vi "Chuck Has Pottable Modules.vi"(8 "error in":errorcluster, 10 "Chuck":i32, 11 "WorkTable in":refnum<class "WorkTable Class.lvclass">=refnum) -> (0 "error out":errorcluster, 2 "Has Pottable Modules":bool, 3 "WorkTable out":refnum<class "WorkTable Class.lvclass">)   [LabVIEW 2017]
uses:
  Shared Components/WorkTable Class/WorkTable Class.lvclass
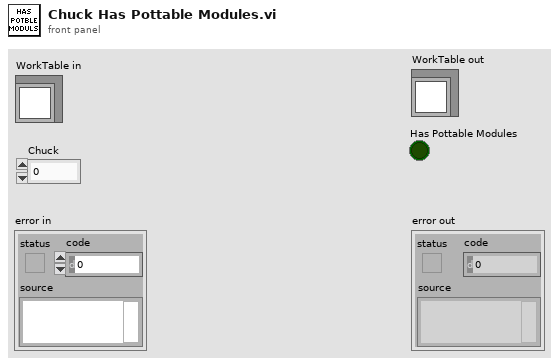
[diagram p1: front panel]
types:
  T1 = typedef "Worktable_Module Slot.ctl" = cluster{"Slot State":enum16{"Empty", "Bare HDI", "Unglued", "Stamped", "PartOnTop", "Weighted", "Unpotted", "Potted"}, "BBM Type":enum16{"None", "BBM", "GlassSlide"}, "HDI Type":enum16{"None", "HDI", "Polyimide"}, "Vacuum Channel":u8, "Location/Orientation BBM":T2, "Location/Orientation HDI":T2, "S/N":string}
  T2 = typedef "Position_Orientation.ctl" = cluster{"Center":refnum<class "Vec3d Class.lvclass">, "Orientation":refnum<class "Orient3d Class.lvclass">}
  T3 = enum16{"Empty", "Unglued", "Stamped", "PartOnTop", "Weighted", "Unpotted", "Potted"}
  T4 = enum16{"Empty", "Bare HDI", "Unglued", "Stamped", "PartOnTop", "Weighted", "Unpotted", "Potted"}
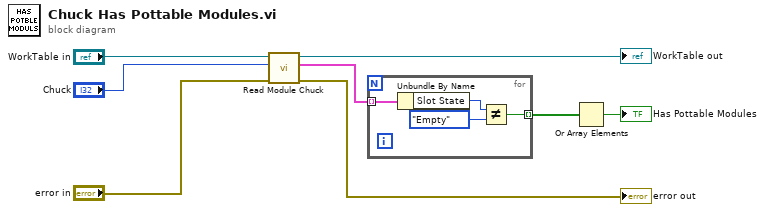
[diagram p0: block diagram]
diagram:
  n1 = call-dynamic "Read Module Chuck.vi"("error in"="error in", "index"="Chuck", "WorkTable in"="WorkTable in") -> ("error out"=→"error out":errorcluster, "Module Slots"=w3:T1[], "WorkTable out"=→"WorkTable out":refnum<class "WorkTable Class.lvclass">)  [unwired: 6 in]
  n2 = for {
    tunnel: w3 -> [w12] mode=indexing
    tunnel: [w9] -> w2 mode=indexing
    n3 = Unbundle By Name(w12) -> ("Slot State"=w11:T4)
    n4 = Not Equal?(x=w11, y=T3."Empty") -> (x != y?=w9:bool)
  }
  n5 = Or Array Elements(Boolean array=w2) -> (logical OR=→"Has Pottable Modules":bool)
